vi "DataProcess_ja.vi"() -> ()   [LabVIEW 2016]
uses:
  <vilib>/Utility/file.llb/Write Delimited Spreadsheet (DBL).vi
  <vilib>/AuZn/auzn custom VIs/AuZnCustomVI.lvlib
panel:
  in  "Output Path":path
  out "Total":i32
  out "Current":i32
  in  "pattern":string
  in  "Path":path
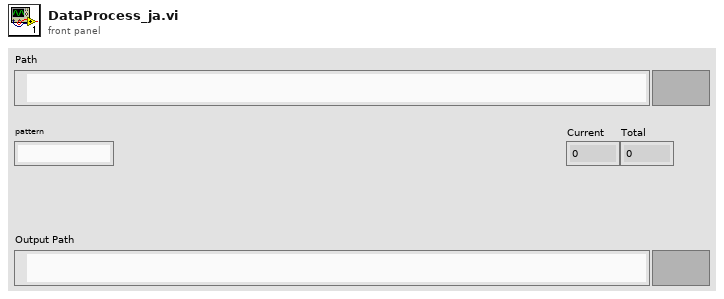
[diagram p1: front panel]
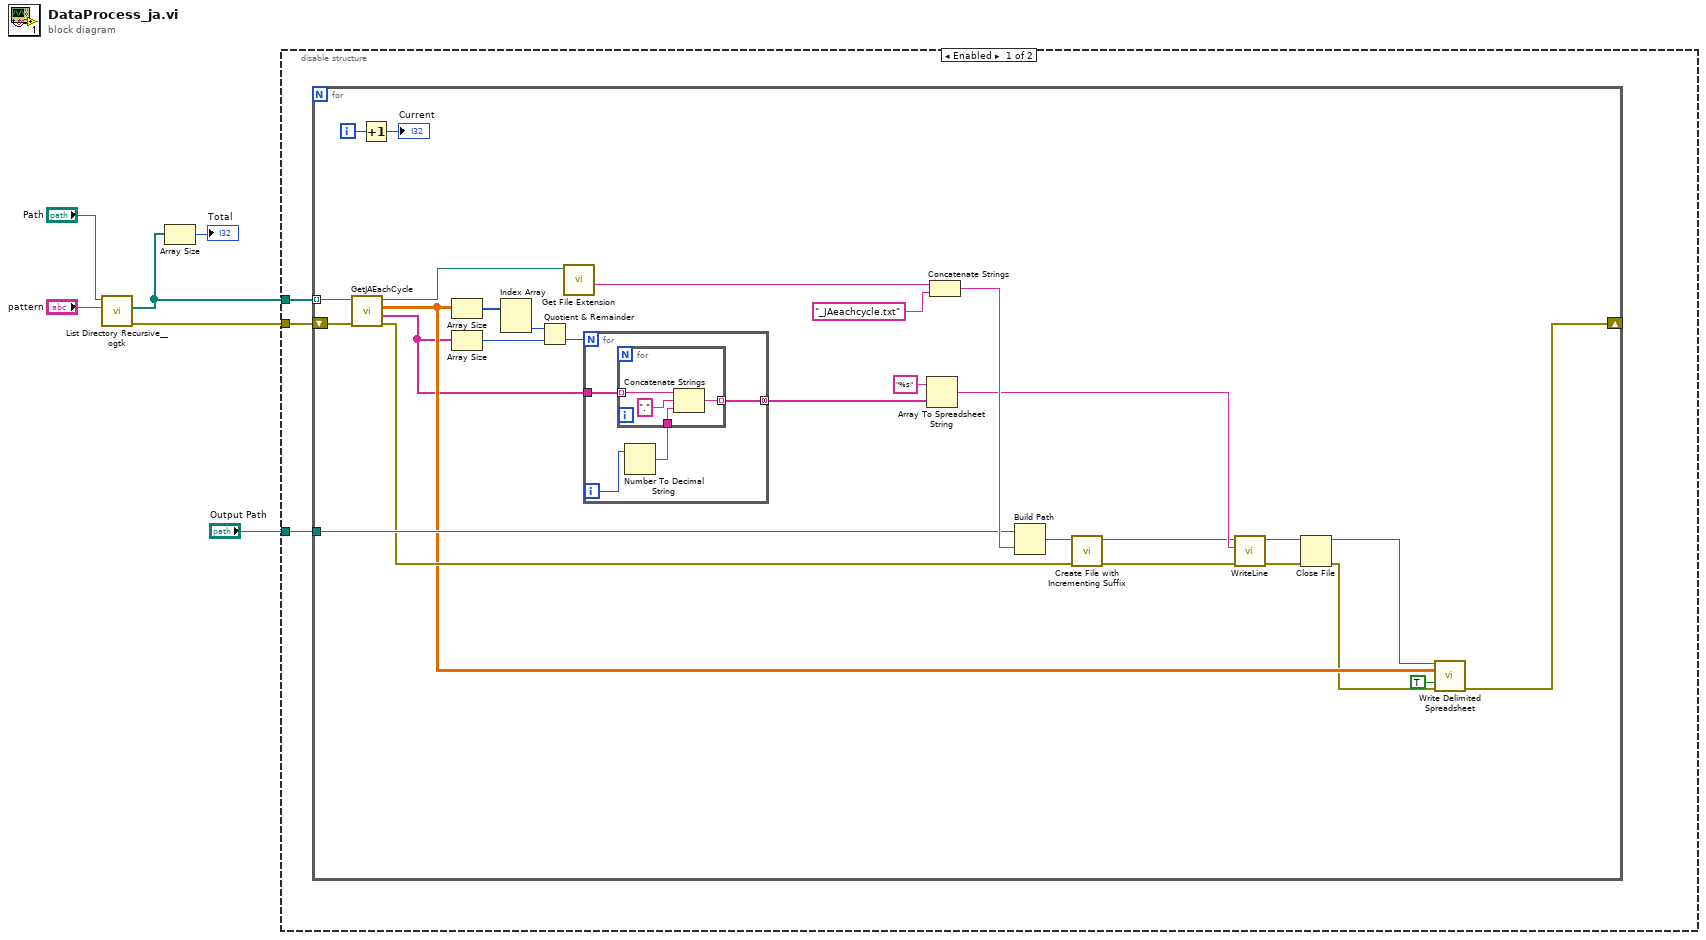
[diagram p0: block diagram]
diagram:
  n1 = call <userlib>:"List Directory Recursive__ogtk.vi"("pattern"="pattern", "Path"="Path") -> ("error out"=w1:errorcluster, "file paths"=w4:path[])  [unwired: 6 in, 2 out]
  n2 = Array Size(array=w4) -> (size(s)=→"Total":i32)
  n3 = disable-structure shown="Enabled" {
    disable-tunnel: w4 -> [w9 _]
    disable-tunnel: "Output Path" -> [w8 _]
    disable-tunnel: w1 -> [w7 _]
    frame Enabled {
      n4 = for {
        tunnel: w9 -> [w31] mode=indexing
        tunnel: w8 -> [w33]
        shift-right: [w32] -> _
        shift-left: w7 -> [w30]
        i -> [w37]
        n5 = call "GetJAEachCycle.vi"("error in (no error)"=w30, "Path"=w31) -> ("error out"=w29:errorcluster, "VarColHeaders"=w24:string[], "JAEachCycle"=w28:dbl[][], "Path dup"=w20:path)  [unwired: 6 in]
        n6 = Increment(x=w37) -> (x+1=→"Current":i32)
        n7 = Array Size(array=w28) -> (size(s)=w27:i32[])
        n8 = Array Size(array=w24) -> (size(s)=w26:i32)
        n9 = Index Array(array=w27) -> (element #2=w18:i32)  [unwired: 2 in, 1 out]
        n10 = Quotient & Remainder(x=w18, y=w26) -> (floor(x/y)=w25:i32)  [unwired: 1 out]
        n11 = call <vilib>:"Get File Extension.vi"("file"=w20) -> ("filename without extension"=w19:string)  [unwired: 6 in, 4 out]
        n12 = for {
          N: w25 -> [_]
          tunnel: w24 -> [w41]
          tunnel: [w38] -> w23 mode=concatenating
          i -> [w40]
          n13 = Number To Decimal String(number=w40) -> (decimal integer string=w39:string)  [unwired: 1 in]
          n14 = for {
            tunnel: w41 -> [w45] mode=indexing
            tunnel: w39 -> [w44]
            tunnel: [w42] -> w38 mode=indexing
            n15 = Concatenate Strings(w45, "." ("string"), w44) -> (w42:string)
          }
        }
        n16 = Array To Spreadsheet String(array=w23, 3:"%s" ("format string")) -> (spreadsheet string=w21:string)  [unwired: 1 in]
        n17 = Concatenate Strings(w19, "_JAeachcycle.txt" ("string")) -> (w35:string)
        n18 = Build Path(base path=w33, name or relative path=w35) -> (appended path=w12:path)
        n19 = call <vilib>:"Create File with Incrementing Suffix.vi"("error in (no error)"=w29, "file path"=w12) -> ("error out"=w10:errorcluster, "refnum out"=w11:refnum<file>)  [unwired: 7 in, 1 out]
        n20 = call <vilib>:"WriteLine.vi"("error in (no error)"=w10, "text"=w21, "refnum in"=w11) -> ("error out"=w14:errorcluster, "refnum out"=w13:refnum<file>)  [unwired: 6 in, 1 out]
        n21 = Close File(refnum=w13, error in=w14) -> (path=w17:path, error out=w16:errorcluster)
        n22 = call-poly <vilib>:"Write Delimited Spreadsheet.vi"("file path (dialog if empty)"=w17, "2D data"=w28, "append to file? (new file:F)"=TRUE ("append to file? (F)"), "error in (no error)"=w16) -> ("error out"=w32:errorcluster)  [unwired: 10 in, 1 out]
      }
    }
    frame Disabled {
    }
  }
